vi "DDAQ-Set-Many.vi"(8 "error in (no error)":errorcluster, 9 "Set Values":string[](array[string]), 10 "SCPI-like Keywords (leave off space, value)":string[](array[string]), 11 "connection ID":refnum<k5>) -> (0 "error out":errorcluster, 3 "connection ID out":refnum<k5>, 4 "Elapsed time, ms (debug)":u32)   [LabVIEW 2020]
panel:
  out "bytes written":i32
  out "Command":string
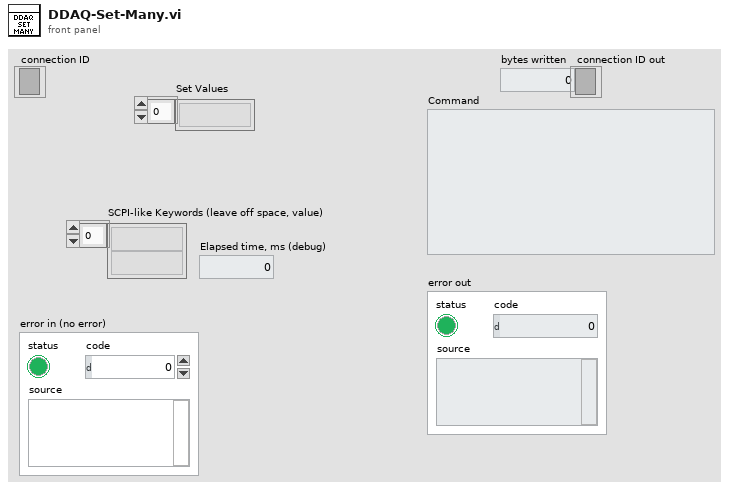
[diagram p1: front panel]
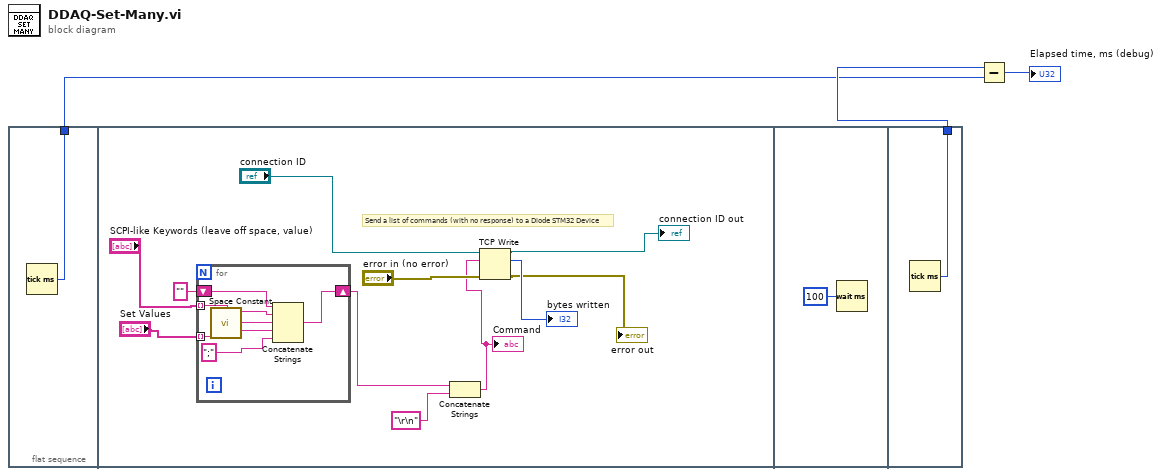
[diagram p0: block diagram]
diagram:
  n1 = flat-sequence {
    tunnel: [w4] -> w2
    tunnel: [w23] -> w3
    frame #0 {
      n2 = Tick Count (ms)() -> (millisecond timer value=w4:u32)
    }
    frame #1 {
      # "Send a list of commands (with no response) to a Diode STM32 Device"
      n3 = for {
        tunnel: "Set Values" -> [w18] mode=indexing
        tunnel: "SCPI-like Keywords (leave off space, value)" -> [w17] mode=indexing
        shift-right: [w21] -> w6
        shift-left: "" -> [w16]
        n4 = call <vilib>:"Space Constant.vi"() -> ("String"=w19:string)
        n5 = Concatenate Strings(w16, w17, w19, w18, ";") -> (w21:string)
      }
      n6 = Concatenate Strings(w6, "\r\n") -> (w5:string)
      "Command" <- w5
      n7 = TCP Write(connection ID="connection ID", data in=w5, error in (no error)="error in (no error)") -> (connection ID out=→"connection ID out":refnum<k5>, bytes written=→"bytes written":i32, error out=→"error out":errorcluster)  [unwired: 1 in]
    }
    frame #2 {
      n8 = Wait (ms)(milliseconds to wait=u32 100) -> ()  [unwired: 1 out]
    }
    frame #3 {
      n9 = Tick Count (ms)() -> (millisecond timer value=w23:u32)
    }
  }
  n10 = Subtract(x=w3, y=w2) -> (x-y=→"Elapsed time, ms (debug)":u32)
